vi "SetChannel.vi"(8 "error in":errorcluster, 9 "index":i32, 10 "T560Channel.lvclass":refnum<class "T560Channel.lvclass">, 11 "T560Session in":refnum<class "T560Session.lvclass">) -> (0 "error out":errorcluster, 3 "T560Session out":refnum<class "T560Session.lvclass">)   [LabVIEW 2020, in "T560Session.lvclass"]
uses:
  T560Session.lvclass
  T560Channel.lvclass
  T560Session.lvclass/T560Session.ctl
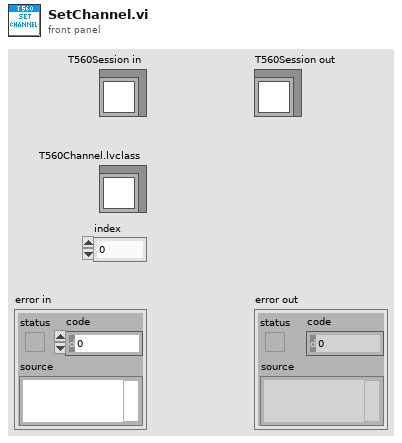
[diagram p1: front panel]
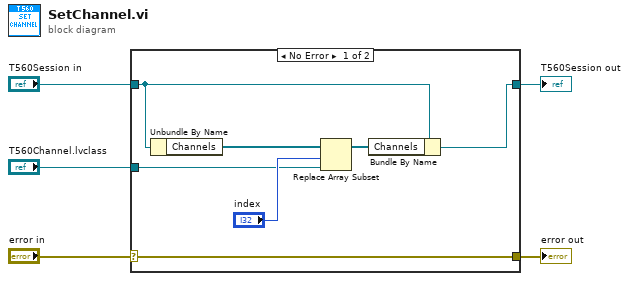
[diagram p0: block diagram]
diagram:
  n1 = case shown="No Error" "error in" {
    selector: "error in" -> [w12 w13]
    tunnel: [w12 w13] -> w4
    tunnel: [w11 w14] -> w2
    tunnel: "T560Session in" -> [w10 w14]
    tunnel: "T560Channel.lvclass" -> [w6 _]
    frame No Error {
      n2 = Unbundle By Name(w10) -> ("Channels"=w9:refnum<class "T560Channel.lvclass">[])
      n3 = Replace Array Subset(array=w9, new element=w6, index="index") -> (w8:refnum<class "T560Channel.lvclass">[])
      n4 = Bundle By Name(cluster=w10, "Channels"=w8) -> (w11:refnum<class "T560Session.lvclass">)
    }
    frame Error {
    }
  }
  "error out" <- w4
  "T560Session out" <- w2
